vi "VoltageControls.vi"() -> ()   [LabVIEW 2017]
uses:
  <vilib>/DAQmx/write.llb/DAQmx Write (Analog DBL 1Chan 1Samp).vi
  VoltageQueue_Global.vi
  MessageQueue/QueueOperations/Enqueue Message (Single).vi
  <vilib>/DAQmx/miscellaneous.llb/DAQmx Fill In Error Info.vi
  MessageQueue/MessageQueue.lvlib
panel:
  in  "DAQmx Task Name":refnum<k21>="AOD_Voltage"
  in  "stop":bool
  in  "Output":bool
  in  "Voltage":dbl min=0.0 max=5.0 step=0.1
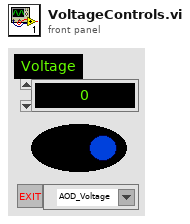
[diagram p1: front panel]
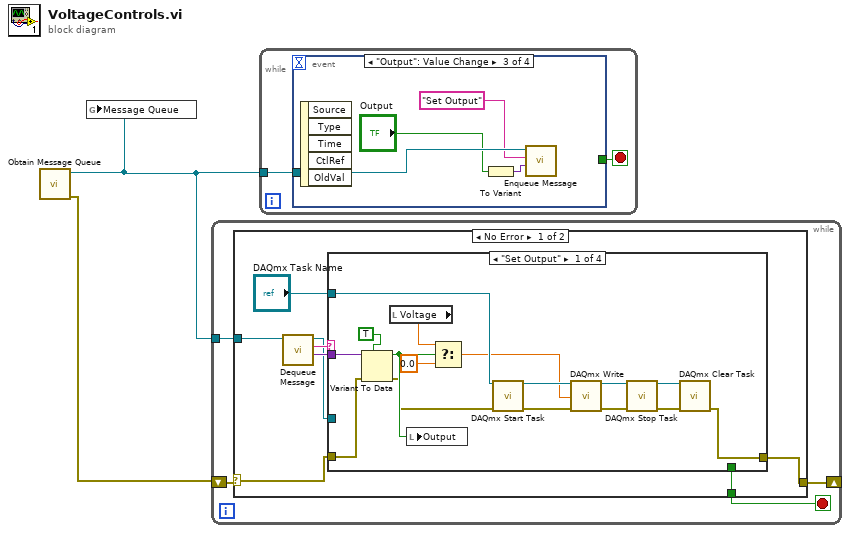
[diagram p0: block diagram]
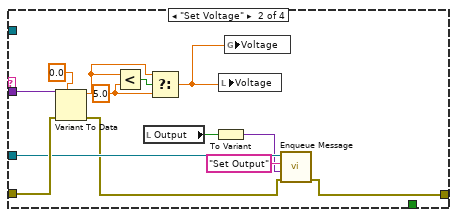
[diagram p2: hidden frame]
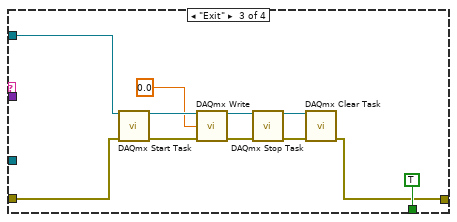
[diagram p3: hidden frame]
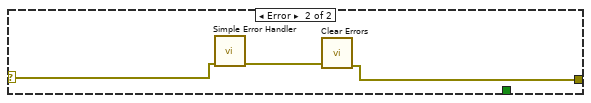
[diagram p5: hidden frame]
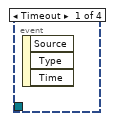
[diagram p6: hidden frame]
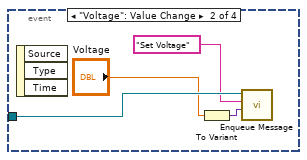
[diagram p7: hidden frame]
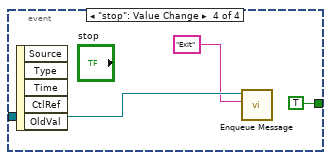
[diagram p8: hidden frame]
diagram:
  n1 = call "Obtain Message Queue.vi"() -> ("error out"=w2:errorcluster, "Message Queue"=w1:refnum<queue>)  [unwired: 10 in]
  n2 = global write "VoltageQueue_Global.vi" "Message Queue"(w1) -> ()
  n3 = while {
    tunnel: w1 -> [w5]
    shift-right: [w4] -> _
    shift-left: w2 -> [w6]
    stop <- w3 stop-if-true
    n4 = case shown="No Error" w6 {
      selector: w6 -> [w11 w56]
      tunnel: w5 -> [w14 _]
      tunnel: [w10 w58] -> w4
      tunnel: [w9 _] -> w3
      frame No Error {
        n5 = call "Dequeue Message.vi"("Message Queue"=w14) -> ("Message Data"=w12:variant, "Message"=w13:string, "dup Message Queue"=w7:refnum<queue>)  [unwired: 7 in, 1 out]
        n6 = case shown="\"Set Output\"" w13 {
          tunnel: w12 -> [w30 w42 _ _]
          tunnel: w11 -> [w28 w41 w45 w55]
          tunnel: [w15 w33 w44 w55] -> w10
          tunnel: [_ _ TRUE _] -> w9
          tunnel: "DAQmx Task Name" -> [w25 _ w47 _]
          tunnel: w7 -> [_ w36 _ _]
          frame "Set Output" {
            n7 = Variant To Data(error in=w28, type=TRUE, Variant=w30) -> (data=w24:bool, error out=w19:errorcluster)
            n8 = local read "Voltage"() -> (w23:dbl)
            n9 = local write "Output"(w24) -> ()
            n10 = Select(t=w23, s=w24, f=0.0) -> (s? t:f=w21:dbl)
            n11 = call <vilib>:"DAQmx Start Task.vi"("task/channels in"=w25, "error in"=w19) -> ("task out"=w27:refnum<k21>, "error out"=w20:errorcluster)  [unwired: 12 in]
            n12 = call-poly <vilib>:"DAQmx Write.vi"("task/channels in"=w27, "data"=w21, "error in"=w20) -> ("task out"=w26:refnum<k21>, "error out"=w18:errorcluster)  [unwired: 10 in, 1 out]
            n13 = call <vilib>:"DAQmx Stop Task.vi"("task/channels in"=w26, "error in"=w18) -> ("task out"=w17:refnum<k21>, "error out"=w16:errorcluster)  [unwired: 12 in]
            n14 = call <vilib>:"DAQmx Clear Task.vi"("task in"=w17, "error in"=w16) -> ("error out"=w15:errorcluster)  [unwired: 13 in]
          }
          frame "Set Voltage" {
            w38 = 5.0 ("y")
            n15 = Variant To Data(error in=w41, type=0.0 ("Voltage"), Variant=w42) -> (data=w40:dbl, error out=w34:errorcluster)
            n16 = Less?(x=w40, y=w38) -> (x < y?=w39:bool)
            n17 = local read "Output"() -> (w32:bool)
            n18 = Select(t=w40, s=w39, f=w38) -> (s? t:f=w37:dbl)
            n19 = To Variant(anything=w32) -> (Variant=w31:variant)
            n20 = local write "Voltage"(w37) -> ()
            n21 = global write "VoltageQueue_Global.vi" "Voltage"(w37) -> ()
            n22 = call-poly "Enqueue Message.vi"("error in (no error)"=w34, "Message Data"=w31, "Message"="Set Output", "Message Queue"=w36) -> ("error out"=w33:errorcluster)  [unwired: 6 in, 1 out]
          }
          frame "Exit" {
            n23 = call <vilib>:"DAQmx Start Task.vi"("task/channels in"=w47, "error in"=w45) -> ("task out"=w48:refnum<k21>, "error out"=w50:errorcluster)  [unwired: 12 in]
            n24 = call-poly <vilib>:"DAQmx Write.vi"("task/channels in"=w48, "data"=0.0, "error in"=w50) -> ("task out"=w49:refnum<k21>, "error out"=w51:errorcluster)  [unwired: 10 in, 1 out]
            n25 = call <vilib>:"DAQmx Stop Task.vi"("task/channels in"=w49, "error in"=w51) -> ("task out"=w52:refnum<k21>, "error out"=w53:errorcluster)  [unwired: 12 in]
            n26 = call <vilib>:"DAQmx Clear Task.vi"("task in"=w52, "error in"=w53) -> ("error out"=w44:errorcluster)  [unwired: 13 in]
          }
          frame Default {
          }
        }
      }
      frame Error {
        n27 = call <vilib>:"Simple Error Handler.vi"("error in (no error)"=w56) -> ("error out"=w57:errorcluster)  [unwired: 4 in, 4 out]
        n28 = call <vilib>:"Clear Errors.vi"("error in (no error)"=w57) -> ("error out"=w58:errorcluster)  [unwired: 5 in, 1 out]
      }
    }
  }
  n29 = while {
    tunnel: w1 -> [w60]
    stop <- w59 stop-if-true
    n30 = event shown="[2] \"Output\": Value Change" {
      selector: _ -> [_ _ _ _]
      dyn-events: _ -> [_ _ _ _]
      timeout: _ -> [_ _ _ _]
      tunnel: w60 -> [_ w64 w68 w71]
      tunnel: [_ _ _ TRUE] -> w59
      event Timeout {
        n31 = event-data() -> ()  [unwired: 1 in, 3 out]
      }
      event "Voltage": Value Change {
        n32 = event-data() -> ()  [unwired: 1 in, 3 out]
        n33 = To Variant(anything="Voltage") -> (Variant=w63:variant)
        n34 = call-poly "Enqueue Message.vi"("Message Data"=w63, "Message"="Set Voltage", "Message Queue"=w64) -> ()  [unwired: 7 in, 2 out]
      }
      event "Output": Value Change {
        n35 = event-data() -> ()  [unwired: 1 in, 5 out]
        n36 = To Variant(anything="Output") -> (Variant=w67:variant)
        n37 = call-poly "Enqueue Message.vi"("Message Data"=w67, "Message"="Set Output", "Message Queue"=w68) -> ()  [unwired: 7 in, 2 out]
      }
      event "stop": Value Change {
        n38 = event-data() -> ()  [unwired: 1 in, 5 out]
        n39 = call-poly "Enqueue Message.vi"("Message"="Exit", "Message Queue"=w71) -> ()  [unwired: 8 in, 2 out]
      }
    }
  }
